vi "Gear Delivery Logging Values.vi"() -> ()   [LabVIEW 2016]
panel:
  out "Gear Chute Position":string
  out "Gear Intake Position":string
  out "Gear Release Position":string
  out "Toggle Intake Rotation and Chute Door":bool
  out "Gear Release":bool
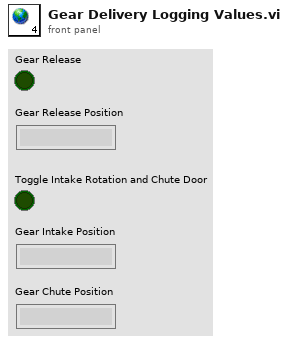
[diagram p1: front panel]
diagram:
